vi "observacao_queued.vi"() -> ()   [LabVIEW 2012, in "Shared_160.lvlib"] (continued)
                n2284 = local read "StatDome"() -> (w2974:string)
                n2285 = Equal?(x=w2974, y="Stopped" ("Status")) -> (x = y?=w2972:bool)
                n2286 = And(x=w2971, y=w2972) -> (x .and. y?=w2970:bool)
                n2287 = case shown="True" w2970 {
                  tunnel: w2969 -> [_ w2975]
                  frame False {
                  }
                  frame True {
                    n2288 = local read "DomeNewPos"() -> (w2982:i32)
                    n2289 = global read "Global_Telescopio.vi" "ErroMaxCup"() -> (w2979:i16)
                    n2290 = global read "Global_Telescopio.vi" "PosCUP"() -> (w2981:i16)
                    n2291 = Multiply(x=w2982, y=w2975) -> (x*y=w2976:i32)
                    n2292 = Subtract(x=w2976, y=w2981) -> (x-y=w2980:i32)
                    n2293 = Absolute Value(x=w2980) -> (abs(x)=w2978:i32)
                    n2294 = Greater?(x=w2978, y=w2979) -> (0:w2977:bool)
                    n2295 = case shown="True" w2977 {
                      tunnel: w2976 -> [_ w2985]
                      frame False {
                      }
                      frame True {
                        # "Desabilita todas Abas"
                        n2296 = local write "DOME"(FALSE) -> ()
                        n2297 = local write "DestCUP"(w2985) -> ()
                        n2298 = property on="Setup, Pointing & Guiding" class="TabCtl (strict)"("Page Selector Visible"=FALSE) -> ()  [unwired: 2 in, 2 out]
                        n2299 = local write "StatDome"("Not Ready" ("Status")) -> ()
                      }
                    }
                  }
                }
              }
              event "BtDomeSTOP": Value Change {
                n2300 = event-data() -> ("NewVal"=w2987:bool)  [unwired: 1 in, 5 out]
                n2301 = case shown="True" w2987 {
                  frame False {
                  }
                  frame True {
                    n2302 = local read "StatDome"() -> (w2988:string)
                    n2303 = case shown="\"Stopped\", Default" w2988 {
                      frame "Stopped", Default {
                      }
                      frame "Moving" {
                        w2989 = u16 4 items=["ZERO", "AH", "DEC", "TUBO", "CUP"] ("Controlador")
                        n2304 = local write "StatDome"("Stopping" ("Status")) -> ()
                        n2305 = call "Monta Comando.vi"("Comando"="PARAR", "Dispositivo"="PROG", "Controlador"=w2989) -> ()  [unwired: 4 in, 3 out]
                      }
                      frame "Not Ready" {
                        n2306 = local write "StatDome"("Stopped" ("Status")) -> ()
                      }
                    }
                  }
                }
              }
              event "BtShutOpen": Value Change {
                n2307 = event-data() -> ("NewVal"=w2995:bool)  [unwired: 1 in, 5 out]
                n2308 = case shown="True" w2995 {
                  frame False {
                  }
                  frame True {
                    n2309 = local read "StatShutter"() -> (w2996:string)
                    n2310 = case shown="\"Closed\"" w2996 {
                      frame "Opened", Default {
                      }
                      frame "Closed" {
                        w2997 = FALSE ("WeakSel")
                        w2998 = FALSE ("Coude")
                        w2999 = T5."Enabled" ("Disabled")
                        n2311 = property on="Coude" class="Bool (strict)"("DisabledEnum"=w2999) -> ()  [unwired: 2 in, 2 out]
                        n2312 = property on="Weak" class="Bool (strict)"("Disabled"=w2999) -> ()  [unwired: 2 in, 2 out]
                        n2313 = local write "StatShutter"("Busy to Open" ("Status")) -> ()
                        n2314 = property on="Medium" class="Bool (strict)"("Disabled"=w2999) -> ()  [unwired: 2 in, 2 out]
                        n2315 = property on="Strong" class="Bool (strict)"("Disabled"=w2999) -> ()  [unwired: 2 in, 2 out]
                        n2316 = local write "WeakSel"(w2997) -> ()
                        n2317 = local write "MediumSel"(w2997) -> ()
                        n2318 = local write "Coude"(w2998) -> ()
                        n2319 = local write "Weak"(w2998) -> ()
                        n2320 = local write "Medium"(w2998) -> ()
                        n2321 = local write "Strong"(w2998) -> ()
                        n2322 = stacked-sequence {
                          frame #0 {
                            w3002 = u16 4 items=["ZERO", "AH", "DEC", "TUBO", "CUP"] ("Controlador")
                            n2323 = call "Monta Comando.vi"("Comando"="DESLIGAR", "Dispositivo"="FLAT_WEAK", "Controlador"=w3002) -> ()  [unwired: 4 in, 3 out]
                          }
                          frame #1 {
                            w3005 = u16 4 items=["ZERO", "AH", "DEC", "TUBO", "CUP"] ("Controlador")
                            n2324 = call "Monta Comando.vi"("Comando"="DESLIGAR", "Dispositivo"="FLAT_LO", "Controlador"=w3005) -> ()  [unwired: 4 in, 3 out]
                          }
                          frame #2 {
                            w3008 = u16 4 items=["ZERO", "AH", "DEC", "TUBO", "CUP"] ("Controlador")
                            n2325 = call "Monta Comando.vi"("Comando"="DESLIGAR", "Dispositivo"="FLAT_HI", "Controlador"=w3008) -> ()  [unwired: 4 in, 3 out]
                          }
                          frame #3 {
                            w3010 = u16 4 items=["ZERO", "AH", "DEC", "TUBO", "CUP"] ("Controlador")
                            n2326 = call "Monta Comando.vi"("Comando"="DESLIGAR", "Dispositivo"="FLAT_COUDE", "Controlador"=w3010) -> ()  [unwired: 4 in, 3 out]
                          }
                        }
                        n2327 = local write "StrongSel"(w2997) -> ()
                        n2328 = local write "CoudeSel"(w2997) -> ()
                      }
                    }
                  }
                }
              }
              event "BtShutClose": Value Change {
                n2329 = event-data() -> ("NewVal"=w3014:bool)  [unwired: 1 in, 5 out]
                n2330 = case shown="True" w3014 {
                  frame False {
                  }
                  frame True {
                    n2331 = stacked-sequence {
                      frame #0 {
                        # "MUDANÇA:\nRemovido CASE que não setava essas\nvariáveis se StatShutter = Closed para\ngarantir fechamento da Trapeira."
                        n2332 = local write "DOME"(FALSE) -> ()
                        n2333 = local write "StatShutter"("Busy to Close" ("Status")) -> ()
                      }
                      frame #1 {
                        # "Escreve no LOG o estado do shutter"
                        # "Timer para escrever no log\ne enviar comando:\nCUP TRAPEIRA PARAR"
                        n2334 = Tick Count (ms)() -> (millisecond timer value=w3017:u32)
                        n2335 = local write "sendCommandShutter"(TRUE ("writeShutterLog")) -> ()
                        n2336 = local write "shutterTimeOld"(w3017) -> ()
                        n2337 = local write "timeStatShutterAlert"(w3017) -> ()
                        n2338 = call "Log_Shutter.vi"("command"=" ", "domeState"="CLOSED " ("command"), "pathLogDomeFile"="C:\\TCS\\LOG\\SHUTTER\\SHUTTER.TXT" ("pathLogFocoString")) -> ()  [unwired: 6 in]
                      }
                    }
                  }
                }
              }
              event "BtParavUp": Value Change {
                n2339 = event-data() -> ("NewVal"=w3022:bool)  [unwired: 1 in, 5 out]
                n2340 = case shown="True" w3022 {
                  frame False {
                  }
                  frame True {
                    w3025 = u16 4 items=["ZERO", "AH", "DEC", "TUBO", "CUP"] ("Controlador")
                    n2341 = call "Monta Comando.vi"("Comando"="SUBIR", "Dispositivo"="PARAVENTO" ("Comando"), "Controlador"=w3025) -> ()  [unwired: 4 in, 3 out]
                  }
                }
              }
              event "BtParavDown": Value Change {
                n2342 = event-data() -> ("NewVal"=w3026:bool)  [unwired: 1 in, 5 out]
                n2343 = case shown="True" w3026 {
                  frame False {
                  }
                  frame True {
                    w3029 = u16 4 items=["ZERO", "AH", "DEC", "TUBO", "CUP"] ("Controlador")
                    n2344 = call "Monta Comando.vi"("Comando"="DESCER", "Dispositivo"="PARAVENTO" ("Comando"), "Controlador"=w3029) -> ()  [unwired: 4 in, 3 out]
                  }
                }
              }
              event "BtParavStop": Value Change {
                n2345 = event-data() -> ("NewVal"=w3030:bool)  [unwired: 1 in, 5 out]
                n2346 = case shown="True" w3030 {
                  frame False {
                  }
                  frame True {
                    w3033 = u16 4 items=["ZERO", "AH", "DEC", "TUBO", "CUP"] ("Controlador")
                    n2347 = call "Monta Comando.vi"("Comando"="PARAR", "Dispositivo"="PARAVENTO" ("Comando"), "Controlador"=w3033) -> ()  [unwired: 4 in, 3 out]
                  }
                }
              }
            }
            n2348 = global read "Global_Telescopio.vi" "PosCUP"() -> (w2877:i16)
            n2349 = local read "RefreshShutterState"() -> (w2878:bool)
            n2350 = call "Bit Status CUP.vi"("NomeStatus"=w2880) -> ("StatBit"=w2879:bool)
            "LedShutter" <- w2879
            n2351 = case shown="\"Stopping\"" w2885 {
              tunnel: w2881 -> [_ w2955 w2962 w2965]
              tunnel: w2882 -> [_ _ _ _]
              frame "", Default {
              }
              frame "Not Ready" {
                n2352 = case shown="False" w2955 {
                  frame False {
                    w2961 = u16 4 items=["ZERO", "AH", "DEC", "TUBO", "CUP"] ("Controlador")
                    n2353 = local read "DestCUP"() -> (w2957:i16)
                    n2354 = local write "StatDome"("Moving" ("Status")) -> ()
                    n2355 = Number To Decimal String(number=w2957) -> (decimal integer string=w2958:string)  [unwired: 1 in]
                    n2356 = call "Monta Comando.vi"("Set Point"=w2958, "Comando"="MOVER", "Dispositivo"="DOMO" ("Comando"), "Controlador"=w2961) -> ()  [unwired: 3 in, 3 out]
                  }
                  frame True {
                  }
                }
              }
              frame "Stopping" {
                n2357 = case shown="False" w2962 {
                  frame False {
                    # "Reabilita Abas"
                    n2358 = property on="Setup, Pointing & Guiding" class="TabCtl (strict)"("Page Selector Visible"=TRUE) -> ()  [unwired: 2 in, 2 out]
                    n2359 = local write "StatDome"("Stopped" ("Status")) -> ()
                  }
                  frame True {
                  }
                }
              }
              frame "Moving" {
                n2360 = case shown="False" w2965 {
                  frame False {
                    # "Reabilita Abas"
                    n2361 = property on="Setup, Pointing & Guiding" class="TabCtl (strict)"("Page Selector Visible"=TRUE) -> ()  [unwired: 2 in, 2 out]
                    n2362 = local write "StatDome"("Stopped" ("Status")) -> ()
                  }
                  frame True {
                  }
                }
              }
            }
            n2363 = case shown="\"Busy to Close\"" w2883 {
              tunnel: w2882 -> [_ _ _ _]
              tunnel: w2881 -> [_ w2938 w2944 _]
              frame "", Default {
              }
              frame "Busy to Open" {
                n2364 = case shown="False" w2938 {
                  frame False {
                    w2942 = u16 4 items=["ZERO", "AH", "DEC", "TUBO", "CUP"] ("Controlador")
                    n2365 = call "TickTimeout.vi"() -> ("msTick"=w2939:u32)  [unwired: 2 in, 2 out]
                    n2366 = local write "TimeoutTrap"(w2939) -> ()
                    n2367 = local write "StatShutter"("Moving" ("Status")) -> ()
                    n2368 = call "Monta Comando.vi"("Comando"="ABRIR", "Dispositivo"="TRAPEIRA" ("Comando"), "Controlador"=w2942) -> ()  [unwired: 4 in, 3 out]
                  }
                  frame True {
                  }
                }
              }
              frame "Busy to Close" {
                n2369 = case shown="False" w2944 {
                  frame False {
                    w2948 = u16 4 items=["ZERO", "AH", "DEC", "TUBO", "CUP"] ("Controlador")
                    n2370 = call "TickTimeout.vi"() -> ("msTick"=w2945:u32)  [unwired: 2 in, 2 out]
                    n2371 = local write "TimeoutTrap"(w2945) -> ()
                    n2372 = local write "StatShutter"("Moving" ("Status")) -> ()
                    n2373 = call "Monta Comando.vi"("Comando"="FECHAR", "Dispositivo"="TRAPEIRA" ("Comando"), "Controlador"=w2948) -> ()  [unwired: 4 in, 3 out]
                  }
                  frame True {
                  }
                }
              }
              frame "Moving" {
                n2374 = local read "TimeoutTrap"() -> (w2950:u32)
                n2375 = call "TickTimeout.vi"("msInicial"=w2950, "msTimeout"=u32 12000) -> ("Timeout"=w2951:bool)  [unwired: 2 out]
                n2376 = case shown="False" w2951 {
                  selector: w2951 -> [w2954 _]
                  frame False {
                    n2377 = Not(x=w2954) -> (.not. x?=w2953:bool)
                    n2378 = local write "RefreshShutterState"(w2953) -> ()
                  }
                  frame True {
                  }
                }
              }
            }
            n2379 = case shown="True" w2878 {
              selector: w2878 -> [_ w2933]
              tunnel: w2879 -> [_ w2934]
              frame False {
              }
              frame True {
                n2380 = Not(x=w2933) -> (.not. x?=→"RefreshShutterState":bool)
                n2381 = Select(t="Opened" ("Status"), s=w2934, f="Closed" ("Status")) -> (s? t:f=w2935:string)
                n2382 = local write "StatShutter"(w2935) -> ()
              }
            }
            n2383 = Divide(x=w2877, y=w2873) -> (x/y=w2888:dbl)
            n2384 = To Word Integer(number=w2888) -> (16bit integer=→"PosCup":i16)
            n2385 = local read "Flag-ShutClose"() -> (w2871:bool)
            n2386 = local read "Flag-ShutOpen"() -> (w2870:bool)
            n2387 = Or(x=w2871, y=w2870) -> (x .or. y?=w2869:bool)
            n2388 = case shown="True" w2869 {
              frame False {
              }
              frame True {
                n2389 = local read "Cont-ShutOpen"() -> (w2910:timestamp)
                n2390 = Get Date/Time In Seconds() -> (seconds since 1Jan1904=w2911:timestamp)
                n2391 = Greater Or Equal?(x=w2911, y=w2910) -> (x >= y?=w2909:bool)
                n2392 = case shown="True" w2909 {
                  frame False {
                  }
                  frame True {
                    w2913 = FALSE ("Flag-ShutClose")
                    # "Reabilita todas Abas"
                    n2393 = local write "Flag-ShutClose"(w2913) -> ()
                    n2394 = local write "Flag-ShutOpen"(w2913) -> ()
                    n2395 = property on="Setup, Pointing & Guiding" class="TabCtl (strict)"("Page Selector Visible"=TRUE) -> ()  [unwired: 2 in, 2 out]
                  }
                }
              }
            }
            n2396 = event shown="[2] \"BtShutOpen\": Value Change" {
              selector: _ -> [_ _ _]
              dyn-events: _ -> [_ _ _]
              timeout: 10 -> [_ _ _]
              event Timeout {
                n2397 = event-data() -> ()  [unwired: 1 in, 2 out]
              }
              event "BtShutClose": Value Change {
                # "Desabilita todas Abas"
                n2398 = event-data() -> ("NewVal"=w2914:bool)  [unwired: 1 in, 4 out]
                n2399 = case shown="True" w2914 {
                  selector: w2914 -> [_ w2919]
                  frame False {
                  }
                  frame True {
                    n2400 = Get Date/Time In Seconds() -> (seconds since 1Jan1904=w2918:timestamp)
                    n2401 = Add(x=w2918, y=10.0) -> (x+y=w2916:timestamp)
                    n2402 = local write "Cont-ShutOpen"(w2916) -> ()
                    n2403 = property on="Setup, Pointing & Guiding" class="TabCtl (strict)"("Page Selector Visible"=FALSE) -> ()  [unwired: 2 in, 2 out]
                    "Flag-ShutClose" <- w2919
                  }
                }
              }
              event "BtShutOpen": Value Change {
                # "Desabilita todas Abas"
                n2404 = event-data() -> ("NewVal"=w2920:bool)  [unwired: 1 in, 4 out]
                n2405 = case shown="True" w2920 {
                  selector: w2920 -> [_ w2921]
                  frame False {
                  }
                  frame True {
                    n2406 = stacked-sequence {
                      tunnel: w2921 -> [w2926 _]
                      frame #0 {
                        n2407 = Get Date/Time In Seconds() -> (seconds since 1Jan1904=w2925:timestamp)
                        n2408 = Add(x=w2925, y=10.0) -> (x+y=→"Cont-ShutOpen":timestamp)
                        n2409 = property on="Setup, Pointing & Guiding" class="TabCtl (strict)"("Page Selector Visible"=FALSE) -> ()  [unwired: 2 in, 2 out]
                        "Flag-ShutOpen" <- w2926
                      }
                      frame #1 {
                        # "Escreve no LOG o estado do shutter"
                        # "Timer para escrever no log\ne enviar comando:\nCUP TRAPEIRA PARAR"
                        n2410 = Tick Count (ms)() -> (millisecond timer value=w2927:u32)
                        n2411 = local write "sendCommandShutter"(TRUE ("writeShutterLog")) -> ()
                        n2412 = local write "timeStatShutterAlert"(w2927) -> ()
                        n2413 = local write "shutterTimeOld"(w2927) -> ()
                        n2414 = call "Log_Shutter.vi"("command"=" ", "domeState"="OPENED " ("command"), "pathLogDomeFile"="C:\\TCS\\LOG\\SHUTTER\\SHUTTER.TXT" ("pathLogFocoString")) -> ()  [unwired: 6 in]
                      }
                    }
                  }
                }
              }
            }
            n2415 = event shown="[3] \"CW\": Mouse Down" {
              selector: _ -> [_ _ _ _ _]
              dyn-events: _ -> [_ _ _ _ _]
              timeout: 100 -> [_ _ _ _ _]
              event Timeout {
                n2416 = event-data() -> ()  [unwired: 1 in, 2 out]
              }
              event "CCW": Mouse Down {
                w2889 = "GIRAR_CCW" ("Comando")
                w2890 = u16 4 items=["ZERO", "AH", "DEC", "TUBO", "CUP"] ("Controlador")
                # "Envia o comando GIRAR"
                n2417 = event-data() -> ()  [unwired: 1 in, 7 out]
                n2418 = local write "Command"(w2889) -> ()
                n2419 = call "Monta Comando.vi"("Comando"=w2889, "Dispositivo"="DOMO" ("Comando"), "Controlador"=w2890) -> ()  [unwired: 4 in, 3 out]
              }
              event "CCW": Mouse Up {
                n2420 = event-data() -> ()  [unwired: 1 in, 7 out]
                n2421 = stacked-sequence {
                  frame #0 {
                    w2892 = "PARAR" ("Comando")
                    w2893 = u16 4 items=["ZERO", "AH", "DEC", "TUBO", "CUP"] ("Controlador")
                    # "Envia o comando PARAR"
                    n2422 = local write "Command"(w2892) -> ()
                    n2423 = call "Monta Comando.vi"("Comando"=w2892, "Dispositivo"="DOMO" ("Comando"), "Controlador"=w2893) -> ()  [unwired: 4 in, 3 out]
                  }
                  frame #1 {
                    n2424 = Wait (ms)(milliseconds to wait=u32 100) -> ()  [unwired: 1 out]
                  }
                  frame #2 {
                    w2896 = "PARAR" ("Comando")
                    w2897 = u16 4 items=["ZERO", "AH", "DEC", "TUBO", "CUP"] ("Controlador")
                    # "Envia o comando PARAR"
                    n2425 = local write "Command"(w2896) -> ()
                    n2426 = call "Monta Comando.vi"("Comando"=w2896, "Dispositivo"="DOMO" ("Comando"), "Controlador"=w2897) -> ()  [unwired: 4 in, 3 out]
                  }
                }
              }
              event "CW": Mouse Down {
                w2899 = "GIRAR_CW" ("Comando")
                w2900 = u16 4 items=["ZERO", "AH", "DEC", "TUBO", "CUP"] ("Controlador")
                # "Envia o comando GIRAR"
                n2427 = event-data() -> ()  [unwired: 1 in, 7 out]
                n2428 = local write "Command"(w2899) -> ()
                n2429 = call "Monta Comando.vi"("Comando"=w2899, "Dispositivo"="DOMO" ("Comando"), "Controlador"=w2900) -> ()  [unwired: 4 in, 3 out]
              }
              event "CW": Mouse Up {
                n2430 = event-data() -> ()  [unwired: 1 in, 7 out]
                n2431 = stacked-sequence {
                  frame #0 {
                    w2902 = "PARAR" ("Comando")
                    w2903 = u16 4 items=["ZERO", "AH", "DEC", "TUBO", "CUP"] ("Controlador")
                    # "Envia o comando PARAR"
                    n2432 = local write "Command"(w2902) -> ()
                    n2433 = call "Monta Comando.vi"("Comando"=w2902, "Dispositivo"="DOMO" ("Comando"), "Controlador"=w2903) -> ()  [unwired: 4 in, 3 out]
                  }
                  frame #1 {
                    n2434 = Wait (ms)(milliseconds to wait=u32 100) -> ()  [unwired: 1 out]
                  }
                  frame #2 {
                    w2906 = "PARAR" ("Comando")
                    w2907 = u16 4 items=["ZERO", "AH", "DEC", "TUBO", "CUP"] ("Controlador")
                    # "Envia o comando PARAR"
                    n2435 = local write "Command"(w2906) -> ()
                    n2436 = call "Monta Comando.vi"("Comando"=w2906, "Dispositivo"="DOMO" ("Comando"), "Controlador"=w2907) -> ()  [unwired: 4 in, 3 out]
                  }
                }
              }
            }
            "Command" <- "" ("Command")
          }
          frame "UTILS " {
            n2437 = stacked-sequence {
              frame #0 {
                # "Acionamento das Abas do\nEspelho\n\nComandos sempre precedidos\nde ESPAÇO\n\nTUBO TAMPAS ESCREVER = 80 80\n\nLigar power geral       08 08\nDesligar power geral  08 00\nLigar System              10 10\nDesligar System         10 00\nPassar para Remoto  20 20\nPassar para Local      20 00\nSel. device central     40 40\nSel. device bowl         40 00\nAction open                80 80\nAction close                80 00"
                n2438 = event shown="[1] \"MODE\": Value Change" {
                  selector: _ -> [_ _ _]
                  dyn-events: _ -> [_ _ _]
                  timeout: 10 -> [_ _ _]
                  event Timeout {
                    n2439 = event-data() -> ()  [unwired: 1 in, 2 out]
                  }
                  event "MODE": Value Change {
                    n2440 = event-data() -> ("NewVal"=w3048:bool)  [unwired: 1 in, 5 out]
                    "LED MODE" <- w3048
                    n2441 = case shown="False" w3048 {
                      frame False {
                        w3053 = u16 3 items=["ZERO", "AH", "DEC", "TUBO", "CUP"] ("Controlador")
                        # "DESABILITA"
                        # "APENAS PASSANDO COMANDO PARA MANETE"
                        # "MODE E GERAL = 0"
                        # "MODE HADSET"
                        n2442 = call "Monta Comando.vi"("Set Point"=" F8 90", "Comando"="ESCREVER", "Dispositivo"="TAMPAS" ("Comando"), "Controlador"=w3053) -> ()  [unwired: 3 in, 3 out]
                        n2443 = property on="ACTION" class="Bool (strict)"("Disabled"=u8 2) -> ()  [unwired: 2 in, 2 out]
                      }
                      frame True {
                        w3058 = u16 3 items=["ZERO", "AH", "DEC", "TUBO", "CUP"] ("Controlador")
                        # "HABILITA"
                        # "APENAS PASSANDO COMOANDO PARA TCSPD"
                        # "MODE E GERAL = 1"
                        # "MODE TCSPD"
                        n2444 = call "Monta Comando.vi"("Set Point"=" 48 48", "Comando"="ESCREVER", "Dispositivo"="TAMPAS" ("Comando"), "Controlador"=w3058) -> ()  [unwired: 3 in, 3 out]
                        n2445 = property on="ACTION" class="Bool (strict)"("Disabled"=u8 0) -> ()  [unwired: 2 in, 2 out]
                      }
                    }
                  }
                  event "ACTION": Value Change {
                    n2446 = event-data() -> ("NewVal"=w3059:bool)  [unwired: 1 in, 5 out]
                    n2447 = case shown="False" w3059 {
                      frame False {
                        # "FECHAR"
                        n2448 = local write "ESTADO FECHAR"("INICIO" ("ESTADO ABRIR")) -> ()
                        n2449 = local write "ESTADO ABRIR"("REPOUSO" ("ESTADO ABRIR")) -> ()
                      }
                      frame True {
                        # "ABRIR"
                        n2450 = local write "ESTADO FECHAR"("REPOUSO" ("ESTADO ABRIR")) -> ()
                        n2451 = local write "ESTADO ABRIR"("INICIO" ("ESTADO ABRIR")) -> ()
                      }
                    }
                  }
                }
                n2452 = Tick Count (ms)() -> (millisecond timer value=w3039:u32)
                n2453 = Greater Or Equal?(x=w3039, y="TIMER TICK") -> (x >= y?=w3035:bool)
                n2454 = And(x=w3035, y=FALSE) -> (x .and. y?=w3036:bool)
                n2455 = case shown="True" w3036 {
                  frame False {
                  }
                  frame True {
                    w3072 = u16 3 items=["ZERO", "AH", "DEC", "TUBO", "CUP", "CASS", "COUDE"] ("Controlador")
                    # "2 SEGUNDOS"
                    n2456 = Tick Count (ms)() -> (millisecond timer value=w3069:u32)
                    n2457 = Add(x=w3069, y=u32 10000) -> (x+y=w3067:u32)
                    n2458 = call "Status_das_Tampas.vi"("Controlador"=w3072, "DISPOSITIVO"="TAMPAS", "Comando"="LER") -> ("Fechado/Aberto"=w3066:bool, "Dispositivo Bacia/Centar"=w3065:bool)  [unwired: 6 in, 5 out]
                    n2459 = local write "TIMER TICK"(w3067) -> ()
                    n2460 = Not(x=w3066) -> (.not. x?=w3064:bool)
                    n2461 = And(x=w3064, y=w3065) -> ()  [unwired: 1 out]
                  }
                }
                n2462 = event shown="[4] \"FLAT-FIELD\": Value Change" {
                  selector: _ -> [_ _ _ _ _ _]
                  dyn-events: _ -> [_ _ _ _ _ _]
                  timeout: 10 -> [_ _ _ _ _ _]
                  event Timeout {
                    n2463 = event-data() -> ()  [unwired: 1 in, 2 out]
                  }
                  event "BtUtilPark": Value Change {
                    n2464 = event-data() -> ("NewVal"=w3073:bool)  [unwired: 1 in, 5 out]
                    n2465 = case shown="True" w3073 {
                      frame False {
                      }
                      frame True {
                        w3076 = u16 4 items=["ZERO", "AH", "DEC", "TUBO", "CUP"] ("Controlador")
                        w3077 = FALSE ("MOUNT")
                        w3080 = 0 ("M_AH")
                        w3081 = u8 2 ("Disabled")
                        w3078 = FALSE ("Page Selector Visible")
                        w3085 = 1 ("M_AH")
                        # "Carrega \nParâmetros \nda Configuração"
                        # "Seta Máq GO"
                        # "Desabilita todas Abas"
                        # "DESABILITA TODOS"
                        n2466 = local write "DOME"(w3078) -> ()
                        n2467 = property on="Setup, Pointing & Guiding" class="TabCtl (strict)"("Page Selector Visible"=w3078) -> ()  [unwired: 2 in, 2 out]
                        n2468 = local write "statAH"(w3080) -> ()
                        n2469 = local write "statCUP"(w3080) -> ()
                        n2470 = local write "statDEC"(w3080) -> ()
                        n2471 = local write "M_DEC"(w3085) -> ()
                        n2472 = local write "M_AH"(w3085) -> ()
                        n2473 = local write "M_CUP"(w3085) -> ()
                        n2474 = global read "Global_Telescopio.vi" "DestDEC"() -> (w3083:dbl)
                        n2475 = global read "Global_Telescopio.vi" "DestCUP"() -> (w3082:i32)
                        n2476 = global read "Global_Telescopio.vi" "DestAH"() -> (w3084:dbl)
                        n2477 = property on="BtUtilPark" class="Bool (strict)"("Disabled"=w3081) -> ()  [unwired: 2 in, 2 out]
                        n2478 = property on="ECASS" class="Bool (strict)"("Disabled"=w3081) -> ()  [unwired: 2 in, 2 out]
                        n2479 = local write "DestAH"(w3084) -> ()
                        n2480 = local write "DestCUP"(w3082) -> ()
                        n2481 = local write "DestDEC"(w3083) -> ()
                        n2482 = global write "Global_Telescopio.vi" "Parking"(TRUE ("Page Selector Visible")) -> ()
                        n2483 = property on="BtUtilZenith" class="Bool (strict)"("Disabled"=w3081) -> ()  [unwired: 2 in, 2 out]
                        n2484 = property on="FLAT-FIELD" class="Bool (strict)"("Disabled"=w3081) -> ()  [unwired: 2 in, 2 out]
                        n2485 = call "Monta Comando.vi"("Comando"="LIGAR", "Dispositivo"="LAMP_CAM" ("Comando"), "Controlador"=w3076) -> ()  [unwired: 4 in, 3 out]
                        n2486 = property on="PROTEÇÃO" class="Bool (strict)"("Disabled"=w3081) -> ()  [unwired: 2 in, 2 out]
                        n2487 = local write "MOUNT"(w3077) -> ()
                        n2488 = local write "GUIDER"(w3077) -> ()
                      }
                    }
                  }
                  event "BtUtilZenith": Value Change {
                    n2489 = event-data() -> ("NewVal"=w3086:bool)  [unwired: 1 in, 5 out]
                    n2490 = case shown="True" w3086 {
                      frame False {
                      }
                      frame True {
                        w3089 = u16 4 items=["ZERO", "AH", "DEC", "TUBO", "CUP"] ("Controlador")
                        w3090 = FALSE ("MOUNT")
                        w3093 = 0 ("M_AH")
                        w3094 = u8 2 ("Disabled")
                        w3092 = FALSE ("Page Selector Visible")
                        w3098 = 1 ("M_AH")
                        # "Seta Máq GO"
                        # "Desabilita todas Abas"
                        # "DESABILITA TODOS"
                        n2491 = local write "M_DEC"(w3098) -> ()
                        n2492 = local write "M_AH"(w3098) -> ()
                        n2493 = local write "M_CUP"(w3098) -> ()
                        n2494 = local write "DOME"(w3092) -> ()
                        n2495 = property on="Setup, Pointing & Guiding" class="TabCtl (strict)"("Page Selector Visible"=w3092) -> ()  [unwired: 2 in, 2 out]
                        n2496 = local write "statAH"(w3093) -> ()
                        n2497 = local write "statCUP"(w3093) -> ()
                        n2498 = local write "statDEC"(w3093) -> ()
                        n2499 = global read "Global_Telescopio.vi" "Telescopio"() -> (w3091:bool)
                        n2500 = property on="BtUtilPark" class="Bool (strict)"("Disabled"=w3094) -> ()  [unwired: 2 in, 2 out]
                        n2501 = property on="ECASS" class="Bool (strict)"("Disabled"=w3094) -> ()  [unwired: 2 in, 2 out]
                        n2502 = case shown="False" w3091 {
                          tunnel: [0.0 ("DestAH") 0.0 ("DestAH")] -> w3097
                          tunnel: [-0.3933 ("DestDEC") -0.3933 ("DestDEC")] -> w3096
                          tunnel: [i16 98 ("DestCUP") i16 80 ("DestCUP")] -> w3095
                          frame False {
                          }
                          frame True {
                          }
                        }
                        n2503 = property on="BtUtilZenith" class="Bool (strict)"("Disabled"=w3094) -> ()  [unwired: 2 in, 2 out]
                        n2504 = property on="FLAT-FIELD" class="Bool (strict)"("Disabled"=w3094) -> ()  [unwired: 2 in, 2 out]
                        n2505 = call "Monta Comando.vi"("Comando"="LIGAR", "Dispositivo"="LAMP_CAM" ("Comando"), "Controlador"=w3089) -> ()  [unwired: 4 in, 3 out]
                        n2506 = local write "DestAH"(w3097) -> ()
                        n2507 = local write "DestCUP"(w3095) -> ()
                        n2508 = local write "DestDEC"(w3096) -> ()
                        n2509 = property on="PROTEÇÃO" class="Bool (strict)"("Disabled"=w3094) -> ()  [unwired: 2 in, 2 out]
                        n2510 = local write "MOUNT"(w3090) -> ()
                        n2511 = local write "GUIDER"(w3090) -> ()
                      }
                    }
                  }
                  event "ECASS": Value Change {
                    n2512 = event-data() -> ("NewVal"=w3105:bool)  [unwired: 1 in, 5 out]
                    n2513 = case shown="True" w3105 {
                      frame False {
                      }
                      frame True {
                        w3108 = u16 4 items=["ZERO", "AH", "DEC", "TUBO", "CUP"] ("Controlador")
                        w3109 = FALSE ("MOUNT")
                        w3112 = 0 ("M_AH")
                        w3113 = u8 2 ("Disabled")
                        w3111 = FALSE ("Page Selector Visible")
                        w3117 = 1 ("M_AH")
                        # "Seta Máq GO"
                        # "Desabilita todas Abas"
                        # "DESABILITA TODOS"
                        n2514 = local write "M_DEC"(w3117) -> ()
                        n2515 = local write "M_AH"(w3117) -> ()
                        n2516 = local write "M_CUP"(w3117) -> ()
                        n2517 = local write "DOME"(w3111) -> ()
                        n2518 = property on="Setup, Pointing & Guiding" class="TabCtl (strict)"("Page Selector Visible"=w3111) -> ()  [unwired: 2 in, 2 out]
                        n2519 = local write "statAH"(w3112) -> ()
                        n2520 = local write "statCUP"(w3112) -> ()
                        n2521 = local write "statDEC"(w3112) -> ()
                        n2522 = global read "Global_Telescopio.vi" "Telescopio"() -> (w3110:bool)
                        n2523 = property on="BtUtilPark" class="Bool (strict)"("Disabled"=w3113) -> ()  [unwired: 2 in, 2 out]
                        n2524 = property on="ECASS" class="Bool (strict)"("Disabled"=w3113) -> ()  [unwired: 2 in, 2 out]
                        n2525 = case shown="False" w3110 {
                          tunnel: [0.0 ("DestAH") 0.0 ("DestAH")] -> w3116
                          tunnel: [0.4 ("DestDEC") 0.4 ("DestDEC")] -> w3115
                          tunnel: [i16 98 ("DestCUP") i16 80 ("DestCUP")] -> w3114
                          frame False {
                          }
                          frame True {
                          }
                        }
                        n2526 = property on="BtUtilZenith" class="Bool (strict)"("Disabled"=w3113) -> ()  [unwired: 2 in, 2 out]
                        n2527 = property on="FLAT-FIELD" class="Bool (strict)"("Disabled"=w3113) -> ()  [unwired: 2 in, 2 out]
                        n2528 = local write "DestAH"(w3116) -> ()
                        n2529 = local write "DestCUP"(w3114) -> ()
                        n2530 = local write "DestDEC"(w3115) -> ()
                        n2531 = call "Monta Comando.vi"("Comando"="LIGAR", "Dispositivo"="LAMP_CAM" ("Comando"), "Controlador"=w3108) -> ()  [unwired: 4 in, 3 out]
                        n2532 = property on="PROTEÇÃO" class="Bool (strict)"("Disabled"=w3113) -> ()  [unwired: 2 in, 2 out]
                        n2533 = local write "GUIDER"(w3109) -> ()
                        n2534 = local write "MOUNT"(w3109) -> ()
                      }
                    }
                  }
                  event "FLAT-FIELD": Value Change {
                    n2535 = event-data() -> ("NewVal"=w3124:bool)  [unwired: 1 in, 5 out]
                    n2536 = case shown="True" w3124 {
                      frame False {
                      }
                      frame True {
                        w3127 = u16 4 items=["ZERO", "AH", "DEC", "TUBO", "CUP"] ("Controlador")
                        w3128 = FALSE ("MOUNT")
                        w3130 = 0 ("M_AH")
                        w3132 = u8 2 ("Disabled")
                        w3131 = FALSE ("Page Selector Visible")
                        w3136 = 1 ("M_AH")
                        # "Seta Máq GO"
                        # "Desabilita todas Abas"
                        # "DESABILITA TODOS"
                        n2537 = local write "M_DEC"(w3136) -> ()
                        n2538 = local write "M_AH"(w3136) -> ()
                        n2539 = local write "M_CUP"(w3136) -> ()
                        n2540 = local write "DOME"(w3131) -> ()
                        n2541 = property on="Setup, Pointing & Guiding" class="TabCtl (strict)"("Page Selector Visible"=w3131) -> ()  [unwired: 2 in, 2 out]
                        n2542 = local write "statAH"(w3130) -> ()
                        n2543 = local write "statCUP"(w3130) -> ()
                        n2544 = local write "statDEC"(w3130) -> ()
                        n2545 = global read "Global_Telescopio.vi" "Telescopio"() -> (w3129:bool)
                        n2546 = property on="BtUtilPark" class="Bool (strict)"("Disabled"=w3132) -> ()  [unwired: 2 in, 2 out]
                        n2547 = property on="ECASS" class="Bool (strict)"("Disabled"=w3132) -> ()  [unwired: 2 in, 2 out]
                        n2548 = case shown="False" w3129 {
                          tunnel: [0.0715 ("DestAH") 0.31416 ("DestAH")] -> w3135
                          tunnel: [0.641 ("DestDEC") -0.39415 ("DestDEC")] -> w3134
                          tunnel: [i16 306 ("DestCUP") i16 133 ("DestCUP")] -> w3133
                          frame False {
                          }
                          frame True {
                          }
                        }
                        n2549 = property on="BtUtilZenith" class="Bool (strict)"("Disabled"=w3132) -> ()  [unwired: 2 in, 2 out]
                        n2550 = property on="FLAT-FIELD" class="Bool (strict)"("Disabled"=w3132) -> ()  [unwired: 2 in, 2 out]
                        n2551 = local write "DestAH"(w3135) -> ()
                        n2552 = local write "DestCUP"(w3133) -> ()
                        n2553 = local write "DestDEC"(w3134) -> ()
                        n2554 = call "Monta Comando.vi"("Comando"="LIGAR", "Dispositivo"="LAMP_CAM" ("Comando"), "Controlador"=w3127) -> ()  [unwired: 4 in, 3 out]
                        n2555 = property on="PROTEÇÃO" class="Bool (strict)"("Disabled"=w3132) -> ()  [unwired: 2 in, 2 out]
                        n2556 = local write "GUIDER"(w3128) -> ()
                        n2557 = local write "MOUNT"(w3128) -> ()
                      }
                    }
                  }
                  event "PROTEÇÃO": Value Change {
                    n2558 = event-data() -> ("NewVal"=w3143:bool)  [unwired: 1 in, 5 out]
                    n2559 = case shown="True" w3143 {
                      frame False {
                      }
                      frame True {
                        w3144 = FALSE ("MOUNT")
                        w3146 = 0 ("M_AH")
                        w3145 = FALSE ("Page Selector Visible")
                        w3148 = u8 2 ("Disabled")
                        # "Seta Máq GO"
                        # "Desabilita todas Abas"
                        # "DESABILITA TODOS"
                        n2560 = local write "DOME"(w3145) -> ()
                        n2561 = property on="Setup, Pointing & Guiding" class="TabCtl (strict)"("Page Selector Visible"=w3145) -> ()  [unwired: 2 in, 2 out]
                        n2562 = local write "statAH"(w3146) -> ()
                        n2563 = local write "statCUP"(w3146) -> ()
                        n2564 = local write "statDEC"(w3146) -> ()
                        n2565 = property on="BtUtilPark" class="Bool (strict)"("Disabled"=w3148) -> ()  [unwired: 2 in, 2 out]
                        n2566 = property on="ECASS" class="Bool (strict)"("Disabled"=w3148) -> ()  [unwired: 2 in, 2 out]
                        n2567 = property on="BtUtilZenith" class="Bool (strict)"("Disabled"=w3148) -> ()  [unwired: 2 in, 2 out]
                        n2568 = property on="FLAT-FIELD" class="Bool (strict)"("Disabled"=w3148) -> ()  [unwired: 2 in, 2 out]
                        n2569 = local write "M_PROT"(1 ("M_PROT")) -> ()
                        n2570 = local write "GUIDER"(w3144) -> ()
                        n2571 = local write "MOUNT"(w3144) -> ()
                        n2572 = property on="PROTEÇÃO" class="Bool (strict)"("Disabled"=w3148) -> ()  [unwired: 2 in, 2 out]
                      }
                    }
                  }
                }
                n2573 = case shown="True" "STOP" {
                  frame False {
                  }
                  frame True {
                    n2574 = stacked-sequence {
                      frame #0 {
                        w3150 = 0 ("estado")
                        # "Zera Máquina de Estado\nPelo Botão STOP"
                        n2575 = property on="Setup, Pointing & Guiding" class="TabCtl (strict)"("Page Selector Visible"=TRUE) -> ()  [unwired: 2 in, 2 out]
                        n2576 = call "Stop.vi"() -> ()  [unwired: 1 in, 1 out]
                        n2577 = local write "Flag Stop"(TRUE ("Flag Stop")) -> ()
                        n2578 = local write "M_AH"(w3150) -> ()
                        n2579 = local write "M_DEC"(w3150) -> ()
                        n2580 = local write "M_CUP"(w3150) -> ()
                        n2581 = local write "M_PROT"(w3150) -> ()
                      }
                      frame #1 {
                        w3152 = FALSE
                        w3153 = u8 0 ("Disabled")
                        # "DESLIGA TODOS"
                        # "HABILITA TODOS"
                        n2582 = local write "BtUtilZenith"(w3152) -> ()
                        n2583 = local write "BtUtilPark"(w3152) -> ()
                        n2584 = local write "FLAT-FIELD"(w3152) -> ()
                        n2585 = local write "PROTEÇÃO"(w3152) -> ()
                        n2586 = local write "ECASS"(w3152) -> ()
                        n2587 = property on="BtUtilPark" class="Bool (strict)"("Disabled"=w3153) -> ()  [unwired: 2 in, 2 out]
                        n2588 = property on="ECASS" class="Bool (strict)"("Disabled"=w3153) -> ()  [unwired: 2 in, 2 out]
                        n2589 = property on="BtUtilZenith" class="Bool (strict)"("Disabled"=w3153) -> ()  [unwired: 2 in, 2 out]
                        n2590 = property on="PROTEÇÃO" class="Bool (strict)"("Disabled"=w3153) -> ()  [unwired: 2 in, 2 out]
                        n2591 = property on="FLAT-FIELD" class="Bool (strict)"("Disabled"=w3153) -> ()  [unwired: 2 in, 2 out]
                      }
                    }
                  }
                }
                n2592 = Compound Arithmetic op=OR("BtUtilPark", "BtUtilZenith", "ECASS", "FLAT-FIELD", "PROTEÇÃO") -> (→"MOVING":bool)
              }
              frame #1 {
                # "MÁQUINAS DE ESTADOS DAS TAMPAS"
                n2593 = case shown="False" "Case Constant\n(See Context Help) 11" {
                  frame False {
                    # "ABRIR"
                    # "FECHAR"
                    n2594 = case shown="\"PIZZA\"" "ESTADO FECHAR" {
                      tunnel: [w3204 w3212 w3223 w3231 w3241 w3249 w3259 "REPOUSO" ("y")] -> w3158
                      frame "INICIO", Default {
                        w3209 = u16 3 items=["ZERO", "AH", "DEC", "TUBO", "CUP"] ("Controlador")
                        # "SELECIONA DISPOSITVO BACIA E\nMANDA FECHAR"
                        # "DISP=1 E PIZZA=1"
                        n2595 = call "Monta Comando.vi"("Set Point"=" A0 A0", "Comando"="ESCREVER", "Dispositivo"="TAMPAS" ("Comando"), "Controlador"=w3209) -> ("Resposta"=w3205:string)  [unwired: 3 in, 2 out]
                        n2596 = Not Equal?(x=w3205, y="TAMPAS OK") -> ()  [unwired: 1 out]
                        n2597 = Tick Count (ms)() -> (millisecond timer value=→"T1 2":u32)
                        n2598 = Select(t="REPOUSO" ("y"), s=FALSE, f="ESPERA 1" ("y")) -> (s? t:f=w3204:string)
                      }
                      frame "ESPERA 1" {
                        # "20 SEGUNDOS"
                        n2599 = local read "T1 2"() -> (w3217:u32)
                        n2600 = Tick Count (ms)() -> (millisecond timer value=w3215:u32)
                        n2601 = Add(x=w3217, y=u32 20000) -> (x+y=w3214:u32)
                        n2602 = Greater?(x=w3215, y=w3214) -> (0:w3211:bool)
                        n2603 = Select(t="PIZZA" ("y"), s=w3211, f="ESPERA 1" ("y")) -> (s? t:f=w3212:string)
                      }
                      frame "PIZZA" {
                        w3228 = u16 3 items=["ZERO", "AH", "DEC", "TUBO", "CUP"] ("Controlador")
                        # "SELECIONA DISP PIZZA\nE MANDA FECHAR"
                        # "PIZZA=1"
                        n2604 = call "Monta Comando.vi"("Set Point"=" 30 10", "Comando"="ESCREVER", "Dispositivo"="TAMPAS" ("Comando"), "Controlador"=w3228) -> ("Resposta"=w3222:string)  [unwired: 3 in, 2 out]
                        n2605 = Tick Count (ms)() -> (millisecond timer value=→"T2 2":u32)
                        n2606 = Not Equal?(x=w3222, y="TAMPAS OK") -> ()  [unwired: 1 out]
                        n2607 = Select(t="REPOUSO" ("y"), s=FALSE, f="PIZZA 2") -> (s? t:f=w3223:string)
                      }
                      frame "PIZZA 2" {
                        w3239 = u16 3 items=["ZERO", "AH", "DEC", "TUBO", "CUP"] ("Controlador")
                        n2608 = call "Monta Comando.vi"("Set Point"=" F8 90", "Comando"="ESCREVER", "Dispositivo"="TAMPAS" ("Comando"), "Controlador"=w3239) -> ("Resposta"=w3234:string)  [unwired: 3 in, 2 out]
                        n2609 = Tick Count (ms)() -> (millisecond timer value=→"T2 3":u32)
                        n2610 = Not Equal?(x=w3234, y="TAMPAS OK") -> ()  [unwired: 1 out]
                        n2611 = Select(t="REPOUSO" ("y"), s=FALSE, f="ESPERA 1A") -> (s? t:f=w3231:string)
                      }
                      frame "ESPERA 1A" {
                        # "2 SEGUNDOS"
                        n2612 = local read "T2 3"() -> (w3244:u32)
                        n2613 = Tick Count (ms)() -> (millisecond timer value=w3246:u32)
                        n2614 = Add(x=w3244, y=u32 2000) -> (x+y=w3247:u32)
                        n2615 = Greater?(x=w3246, y=w3247) -> (0:w3240:bool)
                        n2616 = Select(t="PIZZA 3" ("y"), s=w3240, f="ESPERA 1A" ("y")) -> (s? t:f=w3241:string)
                      }
                      frame "PIZZA 3" {
                        w3257 = u16 3 items=["ZERO", "AH", "DEC", "TUBO", "CUP"] ("Controlador")
                        # "PIZZA=3"
                        n2617 = call "Monta Comando.vi"("Set Point"=" 48 48", "Comando"="ESCREVER", "Dispositivo"="TAMPAS" ("Comando"), "Controlador"=w3257) -> ("Resposta"=w3252:string)  [unwired: 3 in, 2 out]
                        n2618 = Not Equal?(x=w3252, y="TAMPAS OK") -> ()  [unwired: 1 out]
                        n2619 = Select(t="REPOUSO" ("y"), s=FALSE, f="ESPERA 2" ("y")) -> (s? t:f=w3249:string)
                      }
                      frame "ESPERA 2" {
                        # "10 SEGUNDOS"
                        n2620 = local read "T2 2"() -> (w3263:u32)
                        n2621 = Tick Count (ms)() -> (millisecond timer value=w3261:u32)
                        n2622 = Add(x=w3263, y=u32 10000) -> (x+y=w3260:u32)
                        n2623 = Greater?(x=w3261, y=w3260) -> (0:w3258:bool)
                        n2624 = case shown="True" w3258 {
                          frame False {
                          }
                          frame True {
                            n2625 = local write "LED ACTION"(FALSE ("LED ACTION")) -> ()
                          }
                        }
                        n2626 = Select(t="REPOUSO" ("y"), s=w3258, f="ESPERA 2" ("y")) -> (s? t:f=w3259:string)
                      }
                      frame "REPOUSO" {
                      }
                    }
                    n2627 = local write "ESTADO FECHAR"(w3158) -> ()
                    n2628 = case shown="\"INICIO\", Default" "ESTADO ABRIR" {
                      tunnel: [w3163 w3172 w3183 w3190 "REPOUSO" ("y")] -> w3156
                      frame "INICIO", Default {
                        w3169 = u16 3 items=["ZERO", "AH", "DEC", "TUBO", "CUP"] ("Controlador")
                        # "SELECIONA DISPOSITVO PIZZA E\nMANDA ABRIR"
                        # "DISP=0 E PIZZA=0"
                        n2629 = call "Monta Comando.vi"("Set Point"=" 30 00", "Comando"="ESCREVER", "Dispositivo"="TAMPAS" ("Comando"), "Controlador"=w3169) -> ("Resposta"=w3164:string)  [unwired: 3 in, 2 out]
                        n2630 = Not Equal?(x=w3164, y="TAMPAS OK") -> ()  [unwired: 1 out]
                        n2631 = Tick Count (ms)() -> (millisecond timer value=→"T1":u32)
                        n2632 = Select(t="REPOUSO" ("y"), s=FALSE, f="ESPERA 1" ("y")) -> (s? t:f=w3163:string)
                      }
                      frame "ESPERA 1" {
                        # "10 SEGUNDOS"
                        n2633 = local read "T1"() -> (w3177:u32)
                        n2634 = Tick Count (ms)() -> (millisecond timer value=w3175:u32)
                        n2635 = Add(x=w3177, y=u32 10000) -> (x+y=w3174:u32)
                        n2636 = Greater?(x=w3175, y=w3174) -> (0:w3171:bool)
                        n2637 = Select(t="BACIA" ("y"), s=w3171, f="ESPERA 1" ("y")) -> (s? t:f=w3172:string)
                      }
                      frame "BACIA" {
                        w3188 = u16 3 items=["ZERO", "AH", "DEC", "TUBO", "CUP"] ("Controlador")
                        # "SELECIONA DISP BACIA\nE MANDA ABRIR"
                        # "BACIA=0"
                        n2638 = call "Monta Comando.vi"("Set Point"=" A0 20", "Comando"="ESCREVER", "Dispositivo"="TAMPAS" ("Comando"), "Controlador"=w3188) -> ("Resposta"=w3182:string)  [unwired: 3 in, 2 out]
                        n2639 = Tick Count (ms)() -> (millisecond timer value=→"T2":u32)
                        n2640 = Not Equal?(x=w3182, y="TAMPAS OK") -> ()  [unwired: 1 out]
                        n2641 = Select(t="REPOUSO" ("y"), s=FALSE, f="ESPERA 2") -> (s? t:f=w3183:string)
                      }
                      frame "ESPERA 2" {
                        # "25 SEGUNDOS"
                        n2642 = local read "T2"() -> (w3194:u32)
                        n2643 = Tick Count (ms)() -> (millisecond timer value=w3192:u32)
                        n2644 = Add(x=w3194, y=u32 25000) -> (x+y=w3191:u32)
                        n2645 = Greater?(x=w3192, y=w3191) -> (0:w3189:bool)
                        n2646 = case shown="True" w3189 {
                          frame False {
                          }
                          frame True {
                            n2647 = local write "LED ACTION"(TRUE ("LED ACTION")) -> ()
                          }
                        }
                        n2648 = Select(t="REPOUSO" ("y"), s=w3189, f="ESPERA 2" ("y")) -> (s? t:f=w3190:string)
                      }
                      frame "REPOUSO" {
                      }
                    }
                    n2649 = local write "ESTADO ABRIR"(w3156) -> ()
                  }
                  frame True {
                    # "NOVO"
                    # "ABRIR"
                    # "FECHAR"
                    n2650 = local read "ESTADO FECHAR"() -> (w3271:string)
                    n2651 = case shown="\"INICIO\", Default" w3271 {
                      tunnel: [w3336 w3344 w3355 w3363 w3371 "REPOUSO" ("y")] -> w3270
                      frame "INICIO", Default {
                        w3341 = u16 3 items=["ZERO", "AH", "DEC", "TUBO", "CUP"] ("Controlador")
                        # "SELECIONA DISPOSITVO BACIA E\nMANDA FECHAR"
                        n2652 = call "Monta Comando.vi"("Set Point"=" A0 A0", "Comando"="ESCREVER", "Dispositivo"="TAMPAS" ("Comando"), "Controlador"=w3341) -> ("Resposta"=w3337:string)  [unwired: 3 in, 2 out]
                        n2653 = Not Equal?(x=w3337, y="TAMPAS OK") -> ()  [unwired: 1 out]
                        n2654 = Tick Count (ms)() -> (millisecond timer value=→"TF1":u32)
                        n2655 = Select(t="REPOUSO" ("y"), s=FALSE, f="ESPERA1" ("y")) -> (s? t:f=w3336:string)
                      }
                      frame "ESPERA1" {
                        # "20 SEGUNDOS"
                        n2656 = local read "TF1"() -> (w3349:u32)
                        n2657 = Tick Count (ms)() -> (millisecond timer value=w3347:u32)
                        n2658 = Add(x=w3349, y=u32 20000) -> (x+y=w3346:u32)
                        n2659 = Greater?(x=w3347, y=w3346) -> (0:w3343:bool)
                        n2660 = Select(t="PIZZA" ("y"), s=w3343, f="ESPERA1" ("y")) -> (s? t:f=w3344:string)
                      }
                      frame "PIZZA" {
                        w3360 = u16 3 items=["ZERO", "AH", "DEC", "TUBO", "CUP"] ("Controlador")
                        # "PASSA PARA MODO\nHANDSET E PIZZA FECHA"
                        n2661 = call "Monta Comando.vi"("Set Point"=" 48 00", "Comando"="ESCREVER", "Dispositivo"="TAMPAS" ("Comando"), "Controlador"=w3360) -> ("Resposta"=w3354:string)  [unwired: 3 in, 2 out]
                        n2662 = Tick Count (ms)() -> (millisecond timer value=→"TF2":u32)
                        n2663 = Not Equal?(x=w3354, y="TAMPAS OK") -> ()  [unwired: 1 out]
                        n2664 = Select(t="REPOUSO" ("y"), s=FALSE, f="ESPERA2") -> (s? t:f=w3355:string)
                      }
                      frame "ESPERA2" {
                        # "10 SEGUNDOS"
                        n2665 = local read "TF2"() -> (w3361:u32)
                        n2666 = Tick Count (ms)() -> (millisecond timer value=w3367:u32)
                        n2667 = Add(x=w3361, y=u32 10000) -> (x+y=w3368:u32)
                        n2668 = Greater?(x=w3367, y=w3368) -> (0:w3362:bool)
                        n2669 = Select(t="PIZZA3" ("y"), s=w3362, f="ESPERA2" ("y")) -> (s? t:f=w3363:string)
                      }
                      frame "PIZZA3" {
                        w3379 = u16 3 items=["ZERO", "AH", "DEC", "TUBO", "CUP"] ("Controlador")
                        n2670 = case shown="True" "Case Constant\n(See Context Help) 12" {
                          frame False {
                          }
                          frame True {
                            n2671 = local write "LED ACTION"(FALSE ("LED ACTION")) -> ()
                          }
                        }
                        n2672 = call "Monta Comando.vi"("Set Point"=" 48 48", "Comando"="ESCREVER", "Dispositivo"="TAMPAS" ("Comando"), "Controlador"=w3379) -> ("Resposta"=w3374:string)  [unwired: 3 in, 2 out]
                        n2673 = Not Equal?(x=w3374, y="TAMPAS OK") -> ()  [unwired: 1 out]
                        n2674 = Select(t="REPOUSO" ("y"), s=FALSE, f="REPOUSO" ("y")) -> (s? t:f=w3371:string)
                      }
                      frame "REPOUSO" {
                      }
                    }
                    n2675 = local write "ESTADO FECHAR"(w3270) -> ()
                    n2676 = local read "ESTADO ABRIR"() -> (w3269:string)
                    n2677 = case shown="\"INICIO\", Default" w3269 {
                      tunnel: [w3276 w3284 w3292 w3302 w3311 w3324 "REPOUSO" ("y")] -> w3268
                      frame "INICIO", Default {
                        w3282 = u16 3 items=["ZERO", "AH", "DEC", "TUBO", "CUP"] ("Controlador")
                        # "PASSA PARA MODO HANDSET"
                        n2678 = call "Monta Comando.vi"("Set Point"=" F8 00", "Comando"="ESCREVER", "Dispositivo"="TAMPAS" ("Comando"), "Controlador"=w3282) -> ("Resposta"=w3277:string)  [unwired: 3 in, 2 out]
                        n2679 = Not Equal?(x=w3277, y="TAMPAS OK") -> ()  [unwired: 1 out]
                        n2680 = Tick Count (ms)() -> (millisecond timer value=→"TA1":u32)
                        n2681 = Select(t="REPOUSO" ("y"), s=FALSE, f="ESPERA1" ("y")) -> (s? t:f=w3276:string)
                      }
                      frame "ESPERA1" {
                        # "1 SEGUNDO"
                        n2682 = local read "TA1"() -> (w3283:u32)
                        n2683 = Tick Count (ms)() -> (millisecond timer value=w3289:u32)
                        n2684 = Add(x=w3283, y=u32 1000) -> (x+y=w3288:u32)
                        n2685 = Greater?(x=w3289, y=w3288) -> (0:w3286:bool)
                        n2686 = Select(t="ABREPIZZA" ("y"), s=w3286, f="ESPERA1" ("y")) -> (s? t:f=w3284:string)
                      }
                      frame "ABREPIZZA" {
                        w3301 = u16 3 items=["ZERO", "AH", "DEC", "TUBO", "CUP"] ("Controlador")
                        # "MANDA PIZZA ABRIR"
                        n2687 = call "Monta Comando.vi"("Set Point"=" 48 48", "Comando"="ESCREVER", "Dispositivo"="TAMPAS" ("Comando"), "Controlador"=w3301) -> ("Resposta"=w3296:string)  [unwired: 3 in, 2 out]
                        n2688 = Not Equal?(x=w3296, y="TAMPAS OK") -> ()  [unwired: 1 out]
                        n2689 = Tick Count (ms)() -> (millisecond timer value=→"TA2":u32)
                        n2690 = Select(t="ABREPIZZA" ("y"), s=FALSE, f="ESPERA2" ("y")) -> (s? t:f=w3292:string)
                      }
                      frame "ESPERA2" {
                        # "10 SEGUNDOS"
                        n2691 = local read "TA2"() -> (w3303:u32)
                        n2692 = Tick Count (ms)() -> (millisecond timer value=w3308:u32)
                        n2693 = Add(x=w3303, y=u32 10000) -> (x+y=w3307:u32)
                        n2694 = Greater?(x=w3308, y=w3307) -> (0:w3305:bool)
                        n2695 = Select(t="BACIAABRINDO" ("y"), s=w3305, f="ESPERA2" ("y")) -> (s? t:f=w3302:string)
                      }
                      frame "BACIAABRINDO" {
                        w3320 = u16 3 items=["ZERO", "AH", "DEC", "TUBO", "CUP"] ("Controlador")
                        # "BACIA ABRINDO"
                        n2696 = call "Monta Comando.vi"("Set Point"=" A0 20", "Comando"="ESCREVER", "Dispositivo"="TAMPAS" ("Comando"), "Controlador"=w3320) -> ("Resposta"=w3315:string)  [unwired: 3 in, 2 out]
                        n2697 = Not Equal?(x=w3315, y="TAMPAS OK") -> ()  [unwired: 1 out]
                        n2698 = Tick Count (ms)() -> (millisecond timer value=→"TA3":u32)
                        n2699 = Select(t="BACIAABRINDO" ("y"), s=FALSE, f="ESPERA3" ("y")) -> (s? t:f=w3311:string)
                      }
                      frame "ESPERA3" {
                        # "25 SEGUNDOS"
                        n2700 = local read "TA3"() -> (w3322:u32)
                        n2701 = Tick Count (ms)() -> (millisecond timer value=w3327:u32)
                        n2702 = Add(x=w3322, y=u32 25000) -> (x+y=w3326:u32)
